vi "dis_on_test_2.vi"() -> ()   [LabVIEW 2011]
panel:
  out "Last signal with On":dbl=1.0
  in  "Too Low":dbl=1.0
  out "Dark Signal":dbl
  in  "milliseconds to wait":u32=20
  in  "Starting Voltage":dbl=0.1
  in  "Goal Signal":dbl=1.0
  out "Generator Voltage 2":string
  out "Over 2":bool
  out "Signal 2":dbl
  out "Signal":dbl
  out "Over":bool
  out "Generator Voltage":string
  out "Read Back":string
  out "Check":string
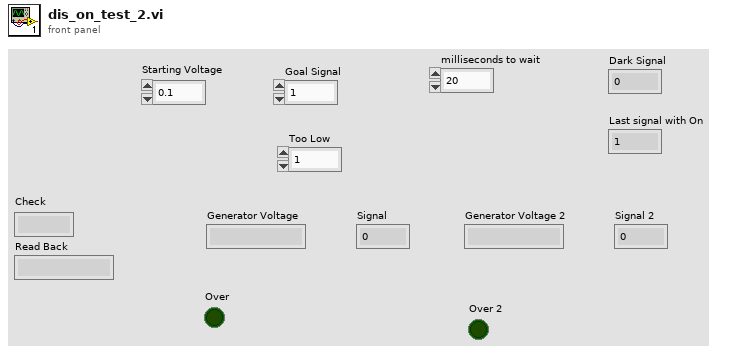
[diagram p1: front panel]
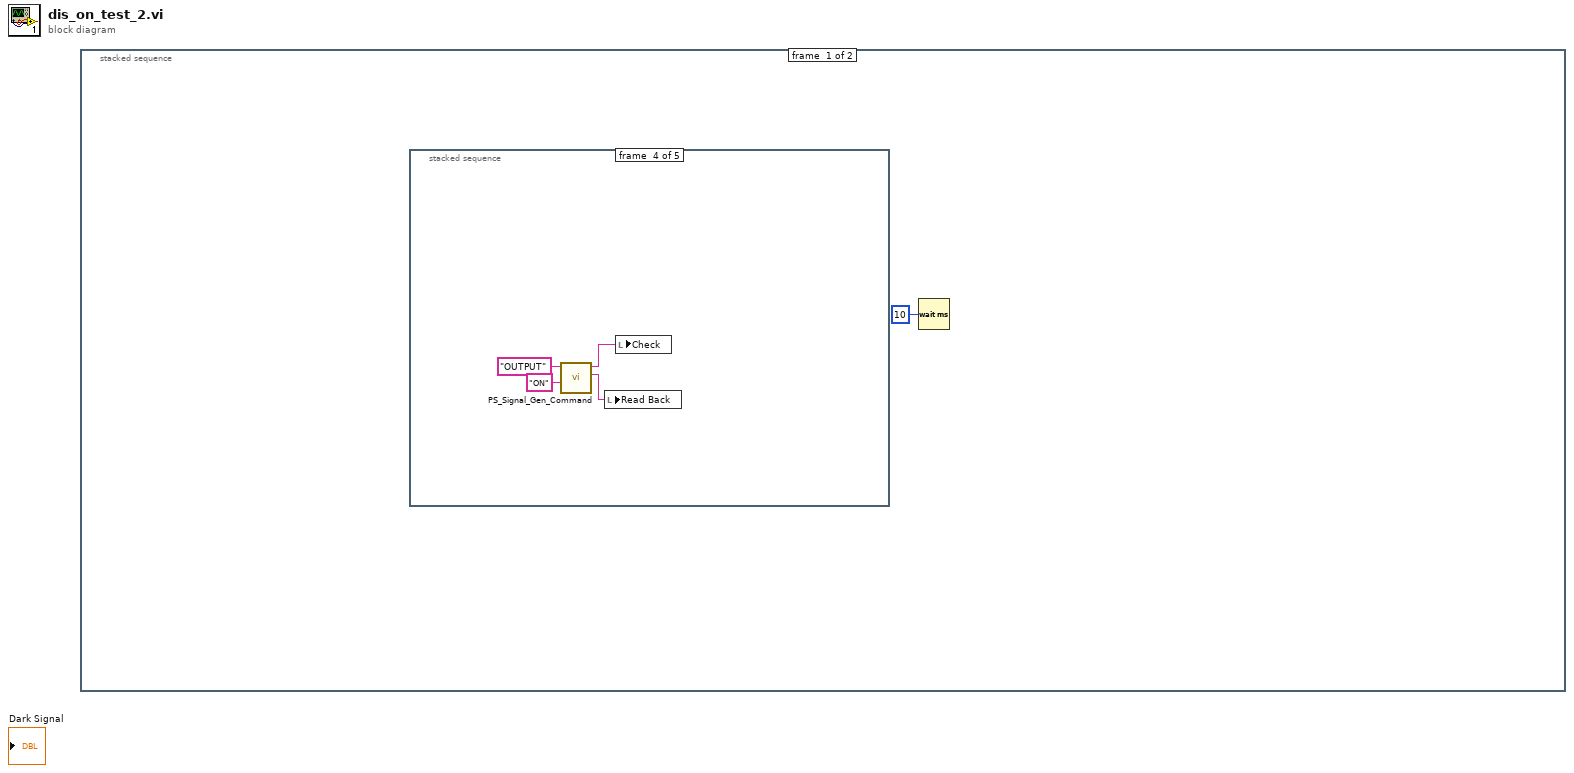
[diagram p0: block diagram]
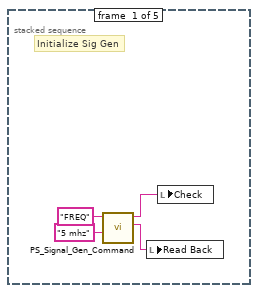
[diagram p2: hidden frame]
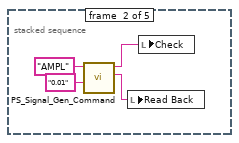
[diagram p3: hidden frame]
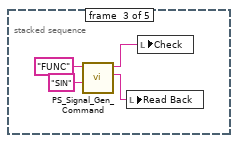
[diagram p4: hidden frame]
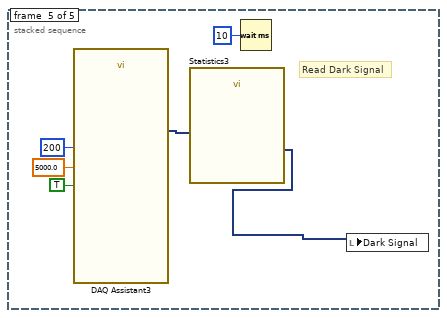
[diagram p5: hidden frame]
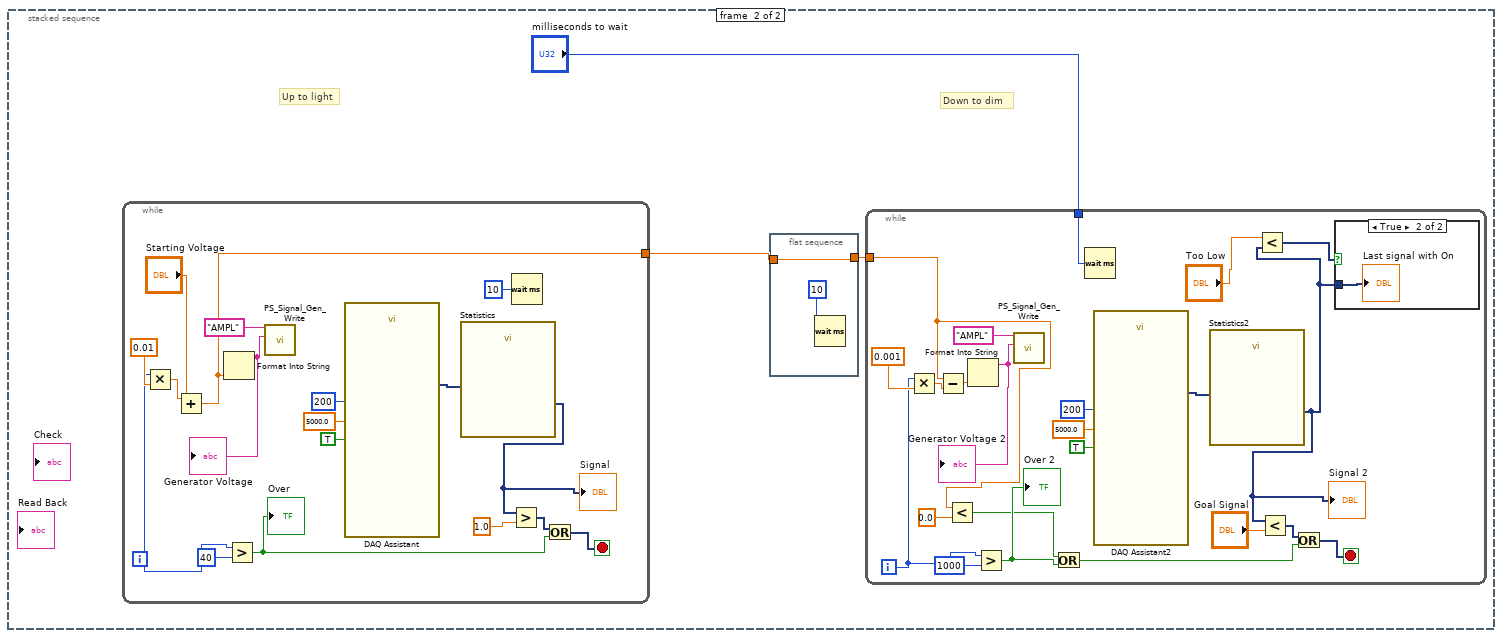
[diagram p6: hidden frame]
diagram:
  n1 = stacked-sequence {
    frame #0 {
      n2 = stacked-sequence {
        frame #0 {
          # "Initialize Sig Gen"
          n3 = call "PS_Signal_Gen_Command.vi"("Value String"="5 mhz", "Command String"="FREQ") -> ("Read Back"=w2:string, "Request String"=w3:string)  [unwired: 7 in, 1 out]
          n4 = local write "Read Back"(w2) -> ()
          n5 = local write "Check"(w3) -> ()
        }
        frame #1 {
          n6 = call "PS_Signal_Gen_Command.vi"("Value String"="0.01", "Command String"="AMPL") -> ("Read Back"=w6:string, "Request String"=w7:string)  [unwired: 7 in, 1 out]
          n7 = local write "Read Back"(w6) -> ()
          n8 = local write "Check"(w7) -> ()
        }
        frame #2 {
          n9 = call "PS_Signal_Gen_Command.vi"("Value String"="SIN", "Command String"="FUNC") -> ("Read Back"=w10:string, "Request String"=w11:string)  [unwired: 7 in, 1 out]
          n10 = local write "Read Back"(w10) -> ()
          n11 = local write "Check"(w11) -> ()
        }
        frame #3 {
          n12 = call "PS_Signal_Gen_Command.vi"("Value String"="ON", "Command String"="OUTPUT") -> ("Read Back"=w14:string, "Request String"=w15:string)  [unwired: 7 in, 1 out]
          n13 = local write "Read Back"(w14) -> ()
          n14 = local write "Check"(w15) -> ()
        }
        frame #4 {
          # "Read Dark Signal"
          n15 = call "DAQ Assistant3"("rate"=5000.0, "number of samples"=200, "stop (F)"=TRUE) -> ("data"=w20:dynamicdata)  [unwired: 13 in, 3 out]
          n16 = call "Statistics3"("Signals"=w20) -> ("Arithmetic Mean"=w18:dynamicdata)  [unwired: 24 in, 2 out]
          n17 = Wait (ms)(milliseconds to wait=u32 10) -> ()  [unwired: 1 out]
          n18 = local write "Dark Signal"(w18) -> ()
        }
      }
      n19 = Wait (ms)(milliseconds to wait=u32 10) -> ()  [unwired: 1 out]
    }
    frame #1 {
      # "Down to dim"
      # "Up to light"
      n20 = while {
        tunnel: [w56] -> w26
        i -> [w69]
        stop <- w63 stop-if-true
        n21 = Multiply(x=w69, y=0.01) -> (x*y=w55:dbl)
        n22 = Add(x=w55, y="Starting Voltage") -> (x+y=w56:dbl)
        n23 = Format Into String(w56) -> (resulting string=w57:string)  [unwired: 3 in, 1 out]
        "Generator Voltage" <- w57
        n24 = Greater?(x=w69, y=40) -> (0:w59:bool)
        "Over" <- w59
        n25 = call "PS_Signal_Gen_Write.vi"("Value String"=w57, "Command String"="AMPL") -> ()  [unwired: 9 in, 1 out]
        n26 = call "DAQ Assistant"("rate"=5000.0, "number of samples"=200, "stop (F)"=TRUE) -> ("data"=w64:dynamicdata)  [unwired: 13 in, 3 out]
        n27 = call "Statistics"("Signals"=w64) -> ("Arithmetic Mean"=w58:dynamicdata)  [unwired: 24 in, 2 out]
        "Signal" <- w58
        n28 = Greater?(x=w58, y=1.0) -> (0:w61:dynamicdata)
        n29 = Wait (ms)(milliseconds to wait=u32 10) -> ()  [unwired: 1 out]
        n30 = Or(x=w61, y=w59) -> (x .or. y?=w63:dynamicdata)
      }
      n31 = flat-sequence {
        tunnel: [w27] -> w25
        tunnel: w26 -> [w27]
        frame #0 {
          n32 = Wait (ms)(milliseconds to wait=u32 10) -> ()  [unwired: 1 out]
        }
      }
      n33 = while {
        tunnel: w25 -> [w34]
        tunnel: "milliseconds to wait" -> [w32]
        i -> [w50]
        stop <- w44 stop-if-true
        n34 = Multiply(x=w50, y=0.001) -> (x*y=w40:dbl)
        n35 = Subtract(x=w34, y=w40) -> (x-y=w39:dbl)
        n36 = Less?(x=w34, y=0.0) -> (x < y?=w36:bool)
        n37 = Format Into String(w39) -> (resulting string=w41:string)  [unwired: 3 in, 1 out]
        "Generator Voltage 2" <- w41
        n38 = Greater?(x=w50, y=1000) -> (0:w37:bool)
        "Over 2" <- w37
        n39 = call "PS_Signal_Gen_Write.vi"("Value String"=w41, "Command String"="AMPL") -> ()  [unwired: 9 in, 1 out]
        n40 = Or(x=w36, y=w37) -> (x .or. y?=w38:bool)
        n41 = Wait (ms)(milliseconds to wait=w32) -> ()  [unwired: 1 out]
        n42 = call "DAQ Assistant2"("rate"=5000.0, "number of samples"=200, "stop (F)"=TRUE) -> ("data"=w45:dynamicdata)  [unwired: 13 in, 3 out]
        n43 = call "Statistics2"("Signals"=w45) -> ("Arithmetic Mean"=w29:dynamicdata)  [unwired: 24 in, 2 out]
        "Signal 2" <- w29
        n44 = Less?(x="Too Low", y=w29) -> (x < y?=w31:dynamicdata)
        n45 = Less?(x=w29, y="Goal Signal") -> (x < y?=w43:dynamicdata)
        n46 = Or(x=w43, y=w38) -> (x .or. y?=w44:dynamicdata)
        n47 = case shown="True" w31 {
          tunnel: w29 -> [_ w52]
          frame False {
          }
          frame True {
            "Last signal with On" <- w52
          }
        }
      }
    }
  }
